vi "Pre Launch Init.vi"(11 "Root Panel Actor in":refnum<class "Root Panel Actor.lvclass">) -> (0 "error out":errorcluster, 3 "Root Panel Actor out":refnum<class "Root Panel Actor.lvclass">)   [LabVIEW 2021, in "Root Panel.lvlib" / "Root Panel Actor.lvclass"]
doc: "Initializes the panel actor. Creates the Panel Helper.\n\n----\nPlease see the following web address for additional documentation and tutorial information:\nhttp://www.mooregoodideas.com/mgi-panel-manager/\n\nAuthor: Derek Trepanier\n\nCopyright (c) 2018, Moore Good Ideas, Inc.\n\nAll rights reserved.\n\nRedistribution and use in source and binary forms, with or without modification, are permitted provided that the following conditions are met:\n\n * Redistributions of source code must retain the above copyright notice, this list of conditions and the following disclaimer.\n * Redistributions in binary form must reproduce the above copyright notice, this list of conditions and the following disclaimer in the documentation and/or other materials provided with the distribution.\n * Neither the name of Moore Good Ideas, Inc. nor the names of its contributors may be used to endorse or promote products derived from this software without specific prior written permission.\n\nTHIS SOFTWARE IS PROVIDED BY THE COPYRIGHT HOLDERS AND CONTRIBUTORS \"AS IS\" AND ANY EXPRESS OR IMPLIED WARRANTIES, INCLUDING, BUT NOT LIMITED TO, THE IMPLIED WARRANTIES OF MERCHANTABILITY AND FITNESS FOR A PARTICULAR PURPOSE ARE DISCLAIMED. IN NO EVENT SHALL THE COPYRIGHT OWNER OR CONTRIBUTORS BE LIABLE FOR ANY DIRECT, INDIRECT, INCIDENTAL, SPECIAL, EXEMPLARY, OR CONSEQUENTIAL DAMAGES (INCLUDING, BUT NOT LIMITED TO, PROCUREMENT OF SUBSTITUTE GOODS OR SERVICES; LOSS OF USE, DATA, OR PROFITS; OR BUSINESS INTERRUPTION) HOWEVER CAUSED AND ON ANY THEORY OF LIABILITY, WHETHER IN CONTRACT, STRICT LIABILITY, OR TORT (INCLUDING NEGLIGENCE OR OTHERWISE) ARISING IN ANY WAY OUT OF THE USE OF THIS SOFTWARE, EVEN IF ADVISED OF THE POSSIBILITY OF SUCH DAMAGE."
uses:
  Root Panel Actor.lvclass
  Typedefs/Paths--enum.ctl
  Appearance Actor/Appearance Actor/Appearance Actor.lvclass
  <vilib>/Thomas ALLIBE/Path Utilities/Path Utilities.lvlib
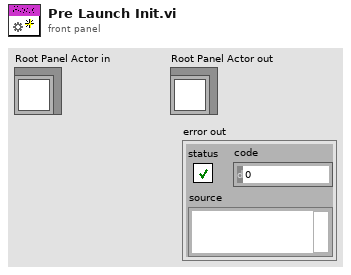
[diagram p1: front panel]
types:
  T1 = typedef "Root Panel.lvlib/Root Panel Actor.lvclass/Paths--enum.ctl" = enum16{"Glbl Config File", "Lang Folder", "Theme Folder"}
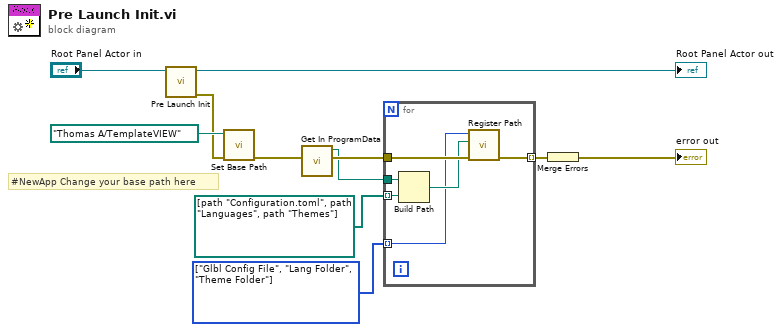
[diagram p0: block diagram]
diagram:
  w3 = T1[] [enum."Glbl Config File", enum."Lang Folder", enum."Theme Folder"] items=["Glbl Config File", "Lang Folder", "Theme Folder"] ("Array")
  # "#NewApp Change your base path here"
  n1 = call-parent "Pre Launch Init.vi"("Appearance Actor in"="Root Panel Actor in") -> ("error out"=w8:errorcluster, "Appearance Actor out"=→"Root Panel Actor out":refnum<class "Root Panel Actor.lvclass">)  [unwired: 9 in]
  n2 = call <vilib>:"Set Base Path.vi"("error in (no error)"=w8, "Base Path"=path "Thomas A/TemplateVIEW") -> ("error out"=w7:errorcluster)  [unwired: 8 in, 1 out]
  n3 = call <vilib>:"Get In ProgramData.vi"("error in (no error)"=w7) -> ("error out"=w6:errorcluster, "Path"=w5:path)  [unwired: 9 in]
  n4 = for {
    tunnel: w6 -> [w17]
    tunnel: w5 -> [w16]
    tunnel: path[] [path "Configuration.toml", path "Languages", path "Themes"] ("name or relative path") -> [w15] mode=indexing
    tunnel: w3 -> [w13] mode=indexing
    tunnel: [w12] -> w2 mode=indexing
    n5 = Build Path(base path=w16, name or relative path=w15) -> (appended path=w14:path)
    n6 = call <vilib>:"Register Path.vi"("error in (no error)"=w17, "Path"=w14, "Key"=w13) -> ("error out"=w12:errorcluster)  [unwired: 6 in, 2 out]
  }
  n7 = Merge Errors(w2) -> (→"error out":errorcluster)
